vi "ClassPanel.vi"(8 "error in (no error)":errorcluster caption="entrée d'erreur (pas d'erreur)", 11 "Spex.lvclass":refnum<class "Spex.lvclass">) -> (0 "error out":errorcluster caption="sortie d'erreur", 3 "Spex.lvclass Out":refnum<class "Spex.lvclass">)   [LabVIEW 2019, in "Spex.lvclass"]
uses:
  Spex.lvclass
  C:/Programmes Labview/LabScanV1A/DevicesClass/BaseDevice/BaseDevice.lvclass
  BaseDevice/Accessor/GetClassEvent.vi
panel:
  in  "MainProgQ":refnum<queue>
  in  "MainProgQEvent":refnum<user-event>
  in  "Acq":bool
  out "Déplacement\nen cours":bool
  in  "MiseAJour":bool
  in  "Stop":bool
  in  "Annuler":bool caption="MiseAJour"
  in  "Position(nm)":dbl=60.0 min=0.1 step=0.1 format="%#.1f"
  out "Init Program":bool
  # "SPEX"
  # "this MUST labeled with class name"
  # "this MUST be present and labeled \"Stop\""
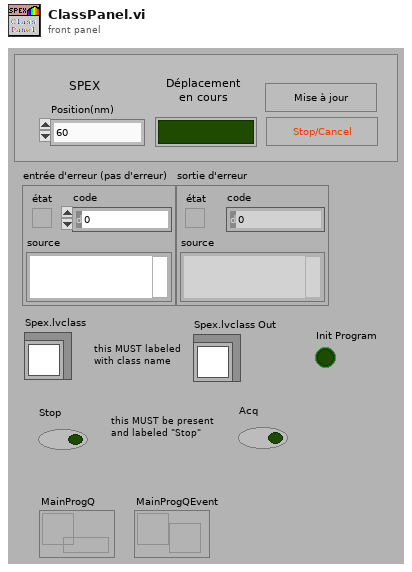
[diagram p1: front panel]
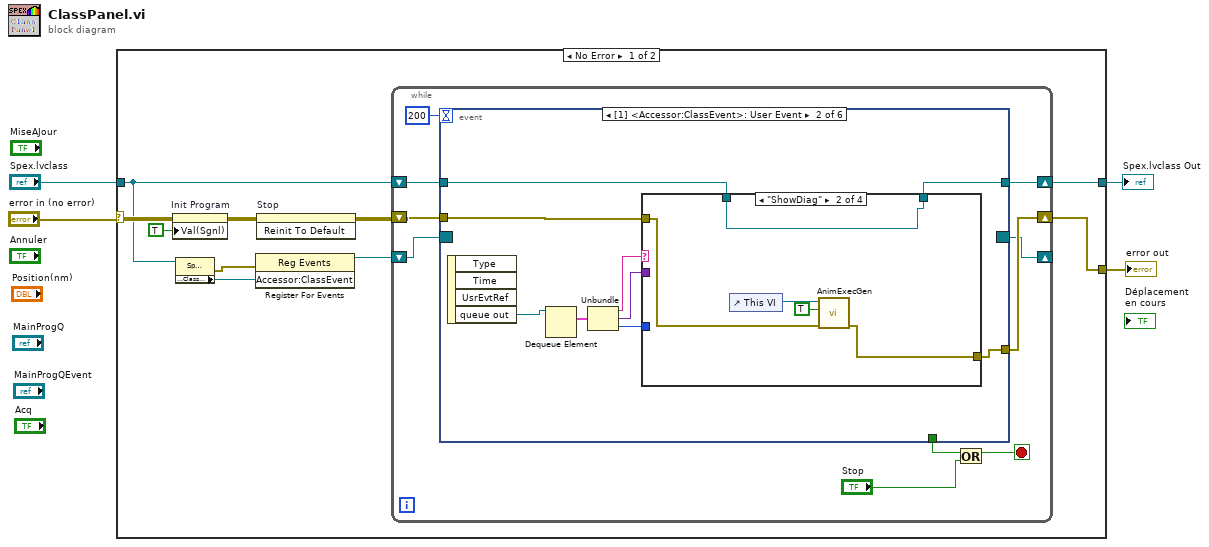
[diagram p0: block diagram]
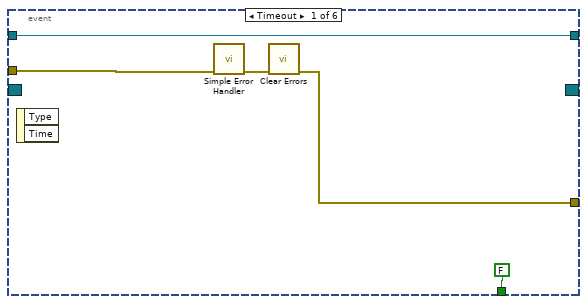
[diagram p2: hidden frame]
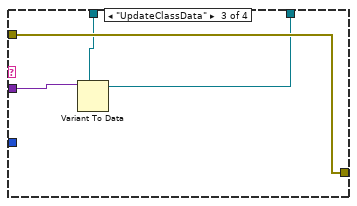
[diagram p4: hidden frame]
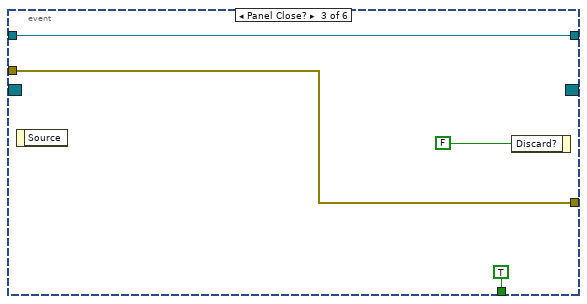
[diagram p6: hidden frame]
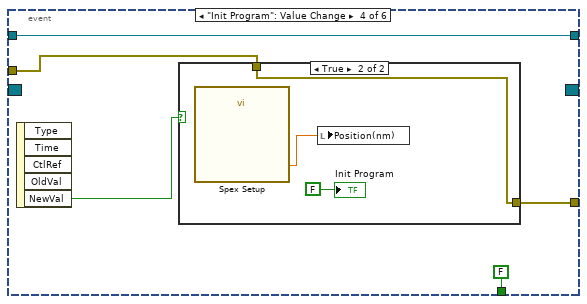
[diagram p7: hidden frame]
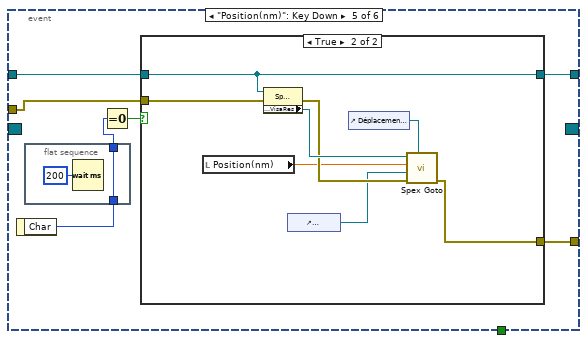
[diagram p9: hidden frame]
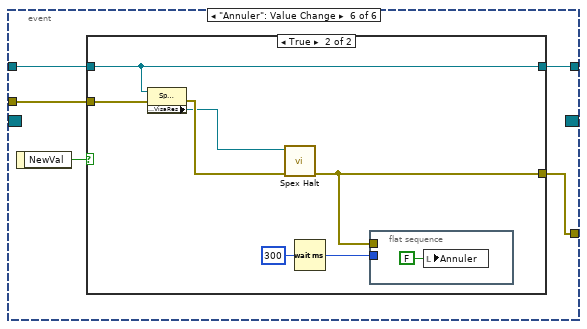
[diagram p11: hidden frame]
diagram:
  n1 = case shown="No Error" "error in (no error)" {
    selector: "error in (no error)" -> [w11 w100]
    tunnel: [w14 w100] -> w3
    tunnel: "Spex.lvclass" -> [w6 w99]
    tunnel: [w12 w99] -> w1
    frame No Error {
      n2 = property on="Init Program" class="Bool (strict)"(error in=w11, "Val(Sgnl)"=TRUE ("Valeur (Signalisation)")) -> (error out=w10:errorcluster)  [unwired: 1 in, 1 out]
      n3 = property class="Spex.lvclass"(reference=w6) -> (error out=w8:errorcluster, "Accessor:ClassEvent"=w7:refnum<user-event>)  [unwired: 1 in, 1 out]
      n4 = register-events(error in=w8, w7) -> (reference out=w5:refnum<event-registration>)  [unwired: 1 in, 1 out]
      n5 = invoke on="Stop" class="Bool (strict)" method="Reinit To Default"(error in=w10) -> (error out=w9:errorcluster)  [unwired: 2 in, 2 out]
      n6 = while {
        shift-right: [w22] -> w14
        shift-left: w9 -> [w23]
        shift-right: [w19] -> w12
        shift-left: w6 -> [w21]
        shift-right: [w15] -> _
        shift-left: w5 -> [w16]
        stop <- w18 stop-if-true
        n7 = event shown="[1] <Accessor:ClassEvent>: User Event" {
          selector: w16 -> [_ _ _ _ _ _]
          dyn-events: [_ _ _ _ _ _] -> w15
          timeout: 200 -> [_ _ _ _ _ _]
          tunnel: w23 -> [w27 w37 w53 w59 w68 w85]
          tunnel: [w25 w31 w53 w58 w65 w84] -> w22
          tunnel: w21 -> [w28 w38 w52 w57 w70 w87]
          tunnel: [FALSE _ TRUE FALSE _ _] -> w20
          tunnel: [w28 w30 w52 w57 w71 w88] -> w19
          event Timeout {
            n8 = event-data() -> ()  [unwired: 1 in, 2 out]
            n9 = call <vilib>:"Simple Error Handler.vi"("error in (no error)"=w27) -> ("error out"=w26:errorcluster)  [unwired: 4 in, 4 out]
            n10 = call <vilib>:"Clear Errors.vi"("error in (no error)"=w26) -> ("error out"=w25:errorcluster)  [unwired: 5 in, 1 out]
          }
          event User Event {
            n11 = event-data() -> ("queue out"=w35:refnum<queue>)  [unwired: 1 in, 3 out]
            n12 = Dequeue Element(queue=w35) -> (element=w36:cluster{"Message":string, "Data":variant, i32})  [unwired: 2 in, 3 out]
            n13 = Unbundle(w36) -> ("Message"=w34:string, "Data"=w33:variant, w32:i32)
            n14 = case shown="\"ShowDiag\"" w34 {
              tunnel: w37 -> [w40 w42 w49 w50]
              tunnel: w33 -> [_ _ w48 _]
              tunnel: w38 -> [w39 w45 w47 w51]
              tunnel: [w39 w45 w46 w51] -> w30
              tunnel: [w40 w41 w49 w50] -> w31
              tunnel: w32 -> [_ _ _ _]
              frame Default {
              }
              frame "ShowDiag" {
                n15 = control-ref of="This VI"() -> (w44:refnum<vi>)
                n16 = call <userlib>:"AnimExecGen.vi"("ErrorIn(No Error)"=w42, "Animer l'exécution ?"=TRUE, "ViRef"=w44) -> ("sortie d'erreur"=w41:errorcluster)  [unwired: 8 in]
              }
              frame "UpdateClassData" {
                n17 = Variant To Data(type=w47, Variant=w48) -> (data=w46:refnum<class "Spex.lvclass">)  [unwired: 1 in, 1 out]
              }
              frame "MeasDone" {
              }
            }
          }
          event Panel Close? {
            n18 = event-data() -> ()  [unwired: 1 in, 1 out]
            n19 = event-data("Discard?"=FALSE ("Rejeter ?")) -> ()  [unwired: 1 in, 1 out]
          }
          event "Init Program": Value Change {
            n20 = event-data() -> ("NewVal"=w60:bool)  [unwired: 1 in, 4 out]
            n21 = case shown="True" w60 {
              tunnel: w59 -> [w61 w63]
              tunnel: [w61 w63] -> w58
              frame False {
              }
              frame True {
                n22 = call "Spex Setup"() -> ("Wavelenght(nm)"=w62:dbl)  [unwired: 17 in, 2 out]
                n23 = local write "Position(nm)"(w62) -> ()
                "Init Program" <- FALSE
              }
            }
          }
          event "Position(nm)": Key Down {
            n24 = event-data() -> ("Char"=w66:i16)  [unwired: 1 in]
            n25 = flat-sequence {
              tunnel: [w72] -> w67
              tunnel: w66 -> [w72]
              frame #0 {
                n26 = Wait (ms)(milliseconds to wait=u32 200 ("attente (ms)")) -> ()  [unwired: 1 out]
              }
            }
            n27 = Equal To 0?(x=w67) -> (x = 0?=w69:bool)
            n28 = case shown="True" w69 {
              tunnel: [w75 w83] -> w71
              tunnel: w70 -> [w75 w83]
              tunnel: w68 -> [w74 w79]
              tunnel: [w74 w76] -> w65
              frame False {
              }
              frame True {
                n29 = local read "Position(nm)"() -> (w78:dbl)
                n30 = property class="Spex.lvclass"(reference=w83, error in=w79) -> (error out=w80:errorcluster, "Accessor:VisaRes"=w82:refnum<visa-resource-name>)  [unwired: 1 out]
                n31 = control-ref of="Position(nm)"() -> (w77:refnum<vi>)
                n32 = control-ref of="Déplacement\nen cours"() -> (w81:refnum<vi>)
                n33 = call <userlib>:"Spex Goto.vi"("Moving Ref"=w81, "error in"=w80, "Lambda Ref"=w77, "Wl(nm)"=w78, "Port"=w82) -> ("error out"=w76:errorcluster)  [unwired: 5 in, 1 out]
              }
            }
          }
          event "Annuler": Value Change {
            n34 = event-data() -> ("NewVal"=w86:bool)  [unwired: 1 in]
            n35 = case shown="True" w86 {
              tunnel: [w89 w97] -> w88
              tunnel: w87 -> [w89 w97]
              tunnel: w85 -> [w90 w96]
              tunnel: [w90 w91] -> w84
              frame False {
              }
              frame True {
                n36 = property class="Spex.lvclass"(reference=w97, error in=w96) -> (error out=w95:errorcluster, "Accessor:VisaRes"=w94:refnum<visa-resource-name>)  [unwired: 1 out]
                n37 = call <userlib>:"Spex Halt.vi"("error in"=w95, "Spex Port"=w94) -> ("error out"=w91:errorcluster)  [unwired: 8 in, 1 out]
                n38 = Wait (ms)(milliseconds to wait=u32 300 ("attente (ms)")) -> (millisecond timer value=w93:u32)
                n39 = flat-sequence {
                  tunnel: w93 -> [_]
                  tunnel: w91 -> [_]
                  frame #0 {
                    n40 = local write "Annuler"(FALSE ("Annuler")) -> ()
                  }
                }
              }
            }
          }
        }
        n41 = Or(x=w20, y="Stop") -> (x .or. y?=w18:bool)
      }
    }
    frame Error {
    }
  }
  "error out" <- w3
  "Spex.lvclass Out" <- w1
